vi "Write Packet.vi"(8 "error in (no error)":errorcluster, 10 "data to write":string, 11 "pcap reference":u32) -> (0 "error out":errorcluster, 3 "pcap reference out":u32)   [LabVIEW 2017, in "lvwpcap.lvlib"]
doc: "This VI reads an ethernet packet. It outputs the packet in the form of a raw string."
uses:
  lvwpcap.lvlib
  LVpcap.dll
panel:
  # "Select Help»Show Context Help and move the cursor over the VI icon to display help for this VI."
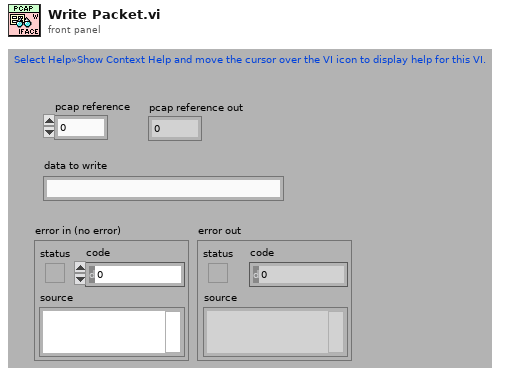
[diagram p1: front panel]
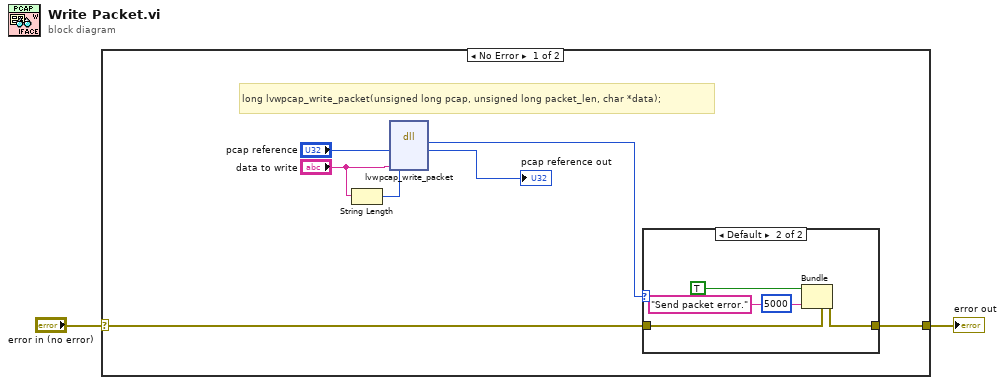
[diagram p0: block diagram]
diagram:
  n1 = case shown="No Error" "error in (no error)" {
    selector: "error in (no error)" -> [w6 w16]
    tunnel: [w9 w16] -> w2
    frame No Error {
      # "long lvwpcap_write_packet(unsigned long pcap, unsigned long packet_len, char *data);"
      n2 = String Length(string="data to write") -> (length=w3:i32)
      n3 = dll-call lib="C:/Users/Michaello/Desktop/MGR NOWEEEEEEEEEEEEEE/MR PROFINET 2017/Lib/WinPcap/LVpcap.dll" fn="lvwpcap_write_packet"("pcap"="pcap reference", "packet_len"=w3, "data"="data to write") -> ("return type"=w8:i32, "pcap"=→"pcap reference out":u32)  [unwired: 5 in, 2 out]
      n4 = case shown="Default" w8 {
        tunnel: w6 -> [w10 w15]
        tunnel: [w10 w13] -> w9
        frame 0 {
        }
        frame Default {
          n5 = Bundle(cluster=w15, "status"=TRUE, "code"=5000, "source"="Send packet error.") -> (w13:errorcluster)
        }
      }
    }
    frame Error {
    }
  }
  "error out" <- w2
